vi "CalStruct SetStrings.vi"(0 "*SerialNumb":string="V12006AD8", 1 "*PcbRevision":string="8", 5 "*ManufactDate":string="02-06-2012    ", 7 "*ManufactLocation":string="NeoTech", 9 "*PcbAssemblyNum":string="EAP0226L50", 11 "error in":errorcluster, 12 "*LastCalLocation":string="SSP") -> (4 "Return Code":i32, 15 "error out":errorcluster)   [LabVIEW 2015]
doc: "This function will update the calibration structure strings in the local EEPROM structure.\n\nint CalStruct_SetStrings (\nchar *SerialNumb,\nchar *ManufactDate,\nchar *ManufactLocation, \nchar *PcbAssemblyNum,\nchar *PcbRevision,\nchar *LastCalDate,\nchar *LastCalLocation);"
uses:
  ScannerDiagDLL.dll
panel:
  out "*LastCalDate":string="04-19-2012  "
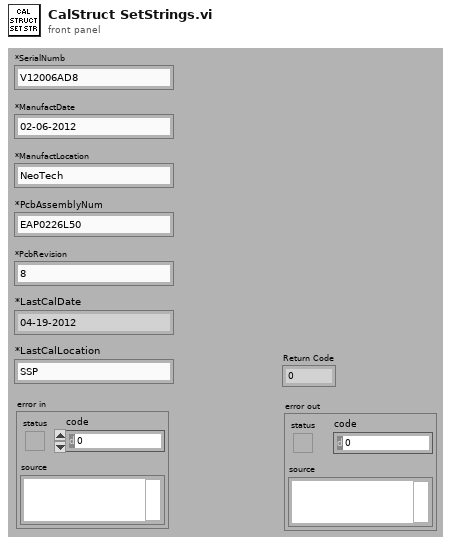
[diagram p1: front panel]
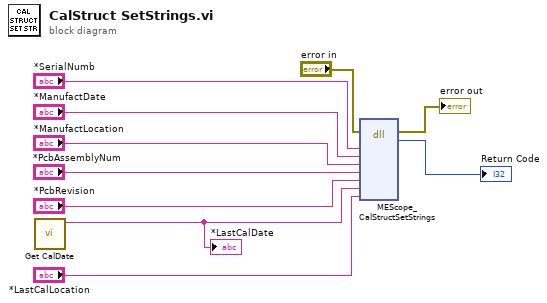
[diagram p0: block diagram]
diagram:
  n1 = call "Get CalDate.vi"() -> ("LastCalDate"=w2:string)  [unwired: 11 in]
  "*LastCalDate" <- w2
  n2 = dll-call lib="C:/SNAPON/ModisEdge/TabletScope/Test Sequence/Code Modules/DLL/ScannerDiagDLL.dll" fn="MEScope_CalStructSetStrings"(error in="error in", "*SerialNumb"="*SerialNumb", "*ManufactDate"="*ManufactDate", "*ManufactLocation"="*ManufactLocation", "*PcbAssemblyNum"="*PcbAssemblyNum", "*PcbRevision"="*PcbRevision", "*LastCalDate"=w2, "*LastCalLocation"="*LastCalLocation") -> (error out=→"error out":errorcluster, "return type"=→"Return Code":i32)  [unwired: 9 in, 1 out]
